vi "Set ErrorList Qref.vi"(8 "error in (no error)":errorcluster, 10 "ErrorList Qref":refnum<queue>, 11 "ErrorHandler in":refnum<class "ErrorHandler.lvclass">) -> (0 "error out":errorcluster, 3 "ErrorHandler out":refnum<class "ErrorHandler.lvclass">)   [LabVIEW 2017, in "ErrorHandler.lvclass"]
doc: "Developed by Kevin Thompson\nkevin@thompsonengineering.net\n\nCopyright 2018\nThompson Engineering, LLC"
uses:
  ErrorHandler.lvclass
  ErrorHandler.lvclass/ErrorHandler.ctl
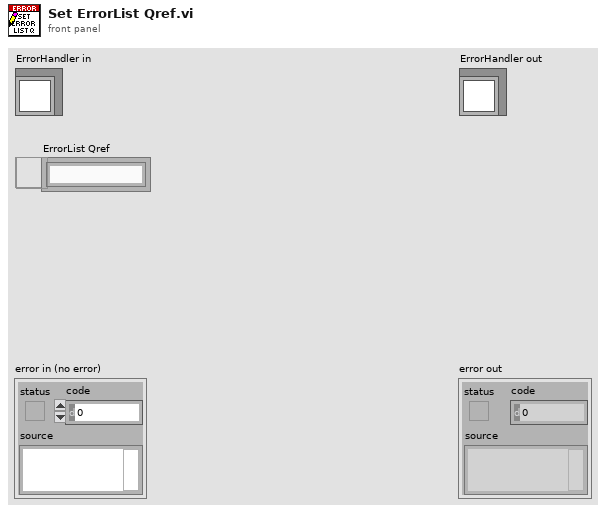
[diagram p1: front panel]
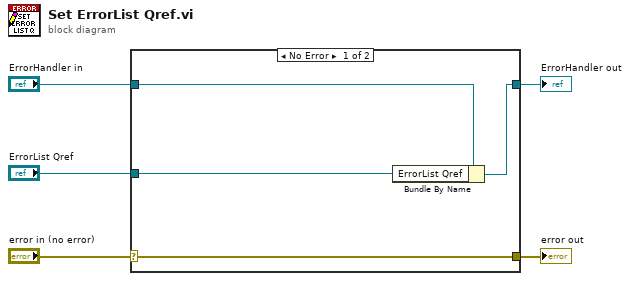
[diagram p0: block diagram]
diagram:
  n1 = case shown="No Error" "error in (no error)" {
    selector: "error in (no error)" -> [w9 w10]
    tunnel: [w9 w10] -> w4
    tunnel: [w7 w11] -> w2
    tunnel: "ErrorHandler in" -> [w8 w11]
    tunnel: "ErrorList Qref" -> [w6 _]
    frame No Error {
      n2 = Bundle By Name(cluster=w8, "ErrorList Qref"=w6) -> (w7:refnum<class "ErrorHandler.lvclass">)
    }
    frame Error {
    }
  }
  "error out" <- w4
  "ErrorHandler out" <- w2
